vi "Drive_Simulated.vi"() -> ()   [LabVIEW 2019]
uses:
  <vilib>/Rock Robotics/WPI/Joystick/WPI_JoystickArcadeMapping.vi
panel:
  out "XY Graph":cluster{"v_linear":dbl[], "v_linear":dbl[]}(graph)
  in  "turn":dbl(slide) scale=-1.0..1.0
  in  "forward":dbl(slide) scale=-1.0..1.0
  in  "Zero XY?":bool
  in  "k_magic":dbl
  in  "b_length":dbl
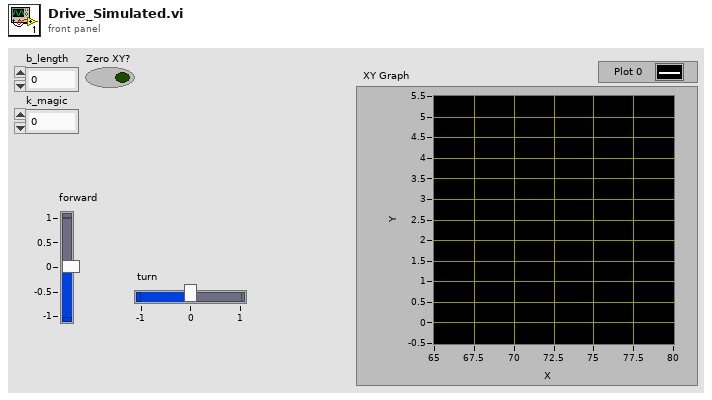
[diagram p1: front panel]
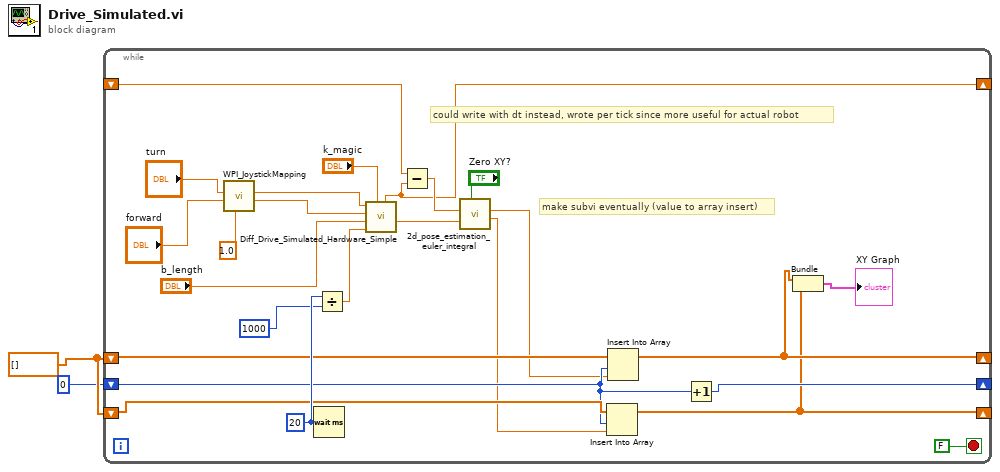
[diagram p0: block diagram]
diagram:
  w2 = dbl[] [] ("v_linear")
  n1 = while {
    shift-right: [w3] -> _
    shift-left: _ -> [w21]
    shift-right: [w5] -> _
    shift-left: w2 -> [w12]
    shift-right: [w4] -> _
    shift-left: w2 -> [w11]
    shift-right: [w9] -> _
    shift-left: u32 0 ("milliseconds to wait") -> [w10]
    stop <- FALSE stop-if-true
    w26 = u32 20 ("milliseconds to wait")
    # "make subvi eventually (value to array insert)"
    # "could write with dt instead, wrote per tick since more useful for actual robot"
    n2 = call-poly <vilib>:"WPI_JoystickMapping.vi"("Max Output"=1.0, "Y axis value"="forward", "X axis value"="turn") -> ("Right Motor Value"=w15:dbl, "Left Motor Value"=w16:dbl)  [unwired: 7 in]
    n3 = Wait (ms)(milliseconds to wait=w26) -> ()  [unwired: 1 out]
    n4 = Divide(x=w26, y=u32 1000 ("milliseconds to wait")) -> (x/y=w24:dbl)
    n5 = call "Diff_Drive_Simulated_Hardware_Simple.vi"("k_magic"="k_magic", "delta_t"=w24, "b_length"="b_length", "%v_bus_right"=w15, "%v_bus_left"=w16) -> ("x_angular"=w19:dbl, "x_linear"=w3:dbl)  [unwired: 1 in, 4 out]
    n6 = Subtract(x=w21, y=w3) -> (x-y=w20:dbl)
    n7 = call "2d_pose_estimation_euler_integral.vi"("Zero XY?"="Zero XY?", "theta(rad)"=w19, "v(per tick)"=w20) -> ("y"=w7:dbl, "x"=w8:dbl)  [unwired: 7 in]
    n8 = Insert Into Array(array=w11, index=w10, new element=w7) -> (w4:dbl[])
    n9 = Insert Into Array(array=w12, index=w10, new element=w8) -> (w5:dbl[])
    n10 = Increment(x=w10) -> (x+1=w9:u32)
    n11 = Bundle("v_linear"=w5, "v_linear"=w4) -> (→"XY Graph":cluster{"v_linear":dbl[], "v_linear":dbl[]})  [unwired: 1 in]
  }
